vi "GetADCTester (SubVI).vi"(8 "error in (no error)":errorcluster, 9 "GetADCTester":T1(ring), 10 "TimeToGet":i32, 11 "VISA Refnum in":refnum<visa-resource-name>) -> (0 "error out":errorcluster, 2 "ADCValOutput Single":dbl, 3 "ADCValOutput Arr":dbl[](array[numeric]))   [LabVIEW 2017]
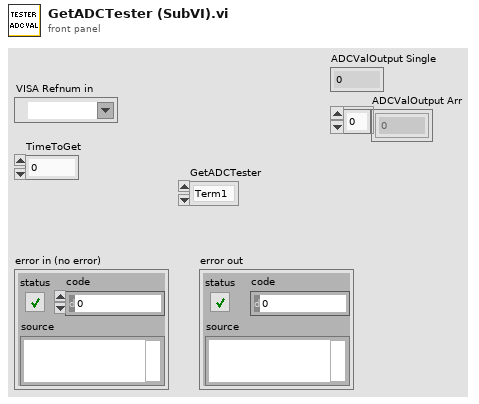
[diagram p1: front panel]
types:
  T1 = enum8{"Term1", "Term2", "Current", "Fan", "TempCPU"}
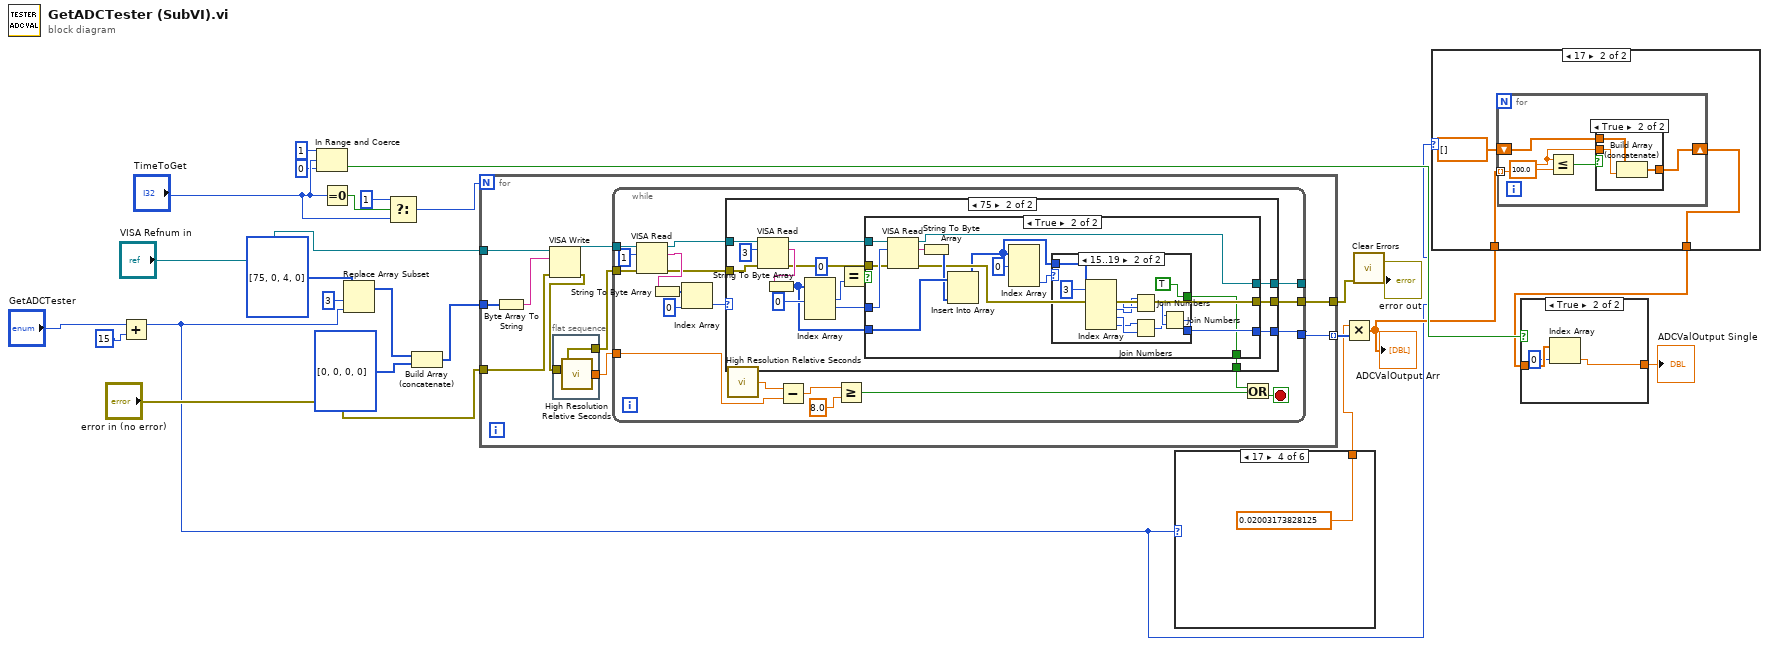
[diagram p0: block diagram]
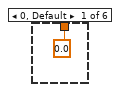
[diagram p4: hidden frame]
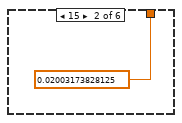
[diagram p5: hidden frame]
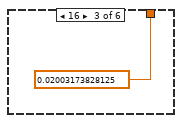
[diagram p6: hidden frame]
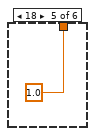
[diagram p7: hidden frame]
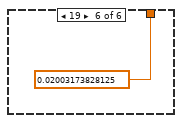
[diagram p8: hidden frame]
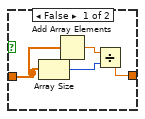
[diagram p9: hidden frame]
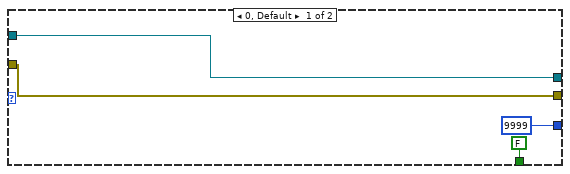
[diagram p10: hidden frame]
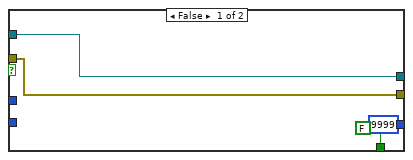
[diagram p11: hidden frame]
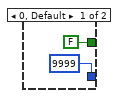
[diagram p12: hidden frame]
diagram:
  n1 = Add(x="GetADCTester", y=u8 15) -> (x+y=w1:u8)
  n2 = In Range and Coerce(upper limit=1, x="TimeToGet", lower limit=0) -> (In Range?=w9:bool)  [unwired: 1 out]
  n3 = Equal To 0?(x="TimeToGet") -> (x = 0?=w22:bool)
  n4 = Replace Array Subset(array=u8[] [75, 0, 4, 0], new element=w1, index=3) -> (w18:u8[])
  n5 = Select(t=1, s=w22, f="TimeToGet") -> (s? t:f=w23:i32)
  n6 = Build Array (concatenate)(w18, u8[] [0, 0, 0, 0]) -> (w19:u8[])
  n7 = for {
    N: w23 -> [_]
    tunnel: "VISA Refnum in" -> [w32]
    tunnel: w19 -> [w31]
    tunnel: [w29] -> w10 mode=indexing
    tunnel: "error in (no error)" -> [w26]
    tunnel: [w30] -> w20
    n8 = Byte Array To String(unsigned byte array=w31) -> (string=w34:string)
    n9 = VISA Write(VISA resource name=w32, write buffer=w34, error in (no error)=w26) -> (VISA resource name out=w33:refnum<visa-resource-name>, error out=w27:errorcluster)  [unwired: 1 out]
    n10 = flat-sequence {
      tunnel: [w36] -> w25
      tunnel: w27 -> [w35]
      tunnel: [w35] -> w28
      frame #0 {
        n11 = call <vilib>:"High Resolution Relative Seconds.vi"() -> ("relative seconds"=w36:dbl)
      }
    }
    n12 = while {
      tunnel: w33 -> [w48]
      tunnel: w28 -> [w47]
      tunnel: [w46] -> _
      tunnel: [w45] -> w30
      tunnel: [w44] -> w29
      tunnel: w25 -> [w41]
      stop <- w43 stop-if-true
      n13 = VISA Read(VISA resource name=w48, byte count=u32 1, error in (no error)=w47) -> (VISA resource name out=w50:refnum<visa-resource-name>, read buffer=w51:string, error out=w49:errorcluster)  [unwired: 1 out]
      n14 = String To Byte Array(string=w51) -> (unsigned byte array=w54:u8[])
      n15 = Index Array(array=w54, index=0) -> (element=w52:u8)
      n16 = case shown="75" w52 {
        tunnel: [w59 w63] -> w45
        tunnel: w50 -> [w58 w72]
        tunnel: w49 -> [w59 w71]
        tunnel: [w58 w64] -> w46
        tunnel: [u32 9999 w61] -> w44
        tunnel: [FALSE w60] -> w42
        frame 0, Default {
        }
        frame 75 {
          n17 = VISA Read(VISA resource name=w72, byte count=u32 3, error in (no error)=w71) -> (VISA resource name out=w67:refnum<visa-resource-name>, read buffer=w75:string, error out=w66:errorcluster)  [unwired: 1 out]
          n18 = String To Byte Array(string=w75) -> (unsigned byte array=w65:u8[])
          n19 = Index Array(array=w65, index #1=0 ("index")) -> (element #1=w70:u8, element #2=w68:u8)  [unwired: 2 in, 1 out]
          n20 = Equal?(x=u8 0, y=w70) -> (x = y?=w69:bool)
          n21 = case shown="True" w69 {
            tunnel: [w78 w85] -> w63
            tunnel: w68 -> [_ w92]
            tunnel: w67 -> [w79 w91]
            tunnel: w66 -> [w78 w90]
            tunnel: w65 -> [_ w89]
            tunnel: [w79 w87] -> w64
            tunnel: [u32 9999 w81] -> w61
            tunnel: [FALSE w80] -> w60
            frame False {
            }
            frame True {
              n22 = VISA Read(VISA resource name=w91, byte count=w92, error in (no error)=w90) -> (VISA resource name out=w87:refnum<visa-resource-name>, read buffer=w86:string, error out=w85:errorcluster)  [unwired: 1 out]
              n23 = String To Byte Array(string=w86) -> (unsigned byte array=w88:u8[])
              n24 = Insert Into Array(array=w89, new element=w88) -> (w82:u8[])  [unwired: 1 in]
              n25 = Index Array(array=w82, index #1=0 ("index")) -> (element #3=w83:u8)  [unwired: 2 in, 2 out]
              n26 = case shown="15..19" w83 {
                tunnel: w82 -> [_ w103]
                tunnel: [u32 9999 w96] -> w81
                tunnel: [FALSE TRUE] -> w80
                frame 0, Default {
                }
                frame 15..19 {
                  n27 = Index Array(array=w103, index #1=3 ("index")) -> (element #1=w102:u8, element #2=w101:u8, element #3=w100:u8, element #4=w99:u8)  [unwired: 3 in]
                  n28 = Join Numbers(hi=w101, lo=w102) -> ((hi.lo)=w98:u16)
                  n29 = Join Numbers(hi=w99, lo=w100) -> ((hi.lo)=w97:u16)
                  n30 = Join Numbers(hi=w97, lo=w98) -> ((hi.lo)=w96:u32)
                }
              }
            }
          }
        }
      }
      n31 = call <vilib>:"High Resolution Relative Seconds.vi"() -> ("relative seconds"=w40:dbl)
      n32 = Subtract(x=w40, y=w41) -> (x-y=w39:dbl)
      n33 = Greater Or Equal?(x=w39, y=8.0) -> (x >= y?=w37:bool)
      n34 = Or(x=w42, y=w37) -> (x .or. y?=w43:bool)
    }
  }
  n35 = case shown="17" w1 {
    tunnel: [0.0 ("x") 0.02003173828125 ("x") 0.02003173828125 ("x") 0.02003173828125 ("x") 1.0 ("x") 0.02003173828125 ("x")] -> w4
    frame 0, Default {
    }
    frame 15 {
    }
    frame 16 {
    }
    frame 17 {
    }
    frame 18 {
    }
    frame 19 {
    }
  }
  n36 = Multiply(x=w4, y=w10) -> (x*y=w3:dbl[])
  "ADCValOutput Arr" <- w3
  n37 = call <vilib>:"Clear Errors.vi"("error in (no error)"=w20) -> ("error out"=→"error out":errorcluster)  [unwired: 5 in, 1 out]
  n38 = case shown="17" w1 {
    tunnel: w3 -> [w111 w114]
    tunnel: [w111 w112] -> w2
    frame 0, Default {
    }
    frame 17 {
      n39 = for {
        tunnel: w114 -> [w117] mode=indexing
        shift-right: [w115] -> w112
        shift-left: dbl[] [] -> [w116]
        n40 = Less Or Equal?(x=w117, y=100.0) -> (x <= y?=w118:bool)
        n41 = case shown="True" w118 {
          tunnel: w117 -> [_ w123]
          tunnel: [w120 w122] -> w115
          tunnel: w116 -> [w120 w121]
          frame False {
          }
          frame True {
            n42 = Build Array (concatenate)(w121, w123) -> (w122:dbl[])
          }
        }
      }
    }
  }
  n43 = case shown="True" w9 {
    tunnel: w2 -> [w127 w130]
    tunnel: [w124 w128] -> w8
    frame False {
      n44 = Array Size(array=w127) -> (size(s)=w125:i32)
      n45 = Add Array Elements(numeric array=w127) -> (sum=w126:dbl)
      n46 = Divide(x=w126, y=w125) -> (x/y=w124:dbl)
    }
    frame True {
      n47 = Index Array(array=w130, index=0) -> (element=w128:dbl)
    }
  }
  "ADCValOutput Single" <- w8
